vi "SeCrTs-RD DI Indexing dis.vi"() -> ()   [LabVIEW 2022 SP3]
panel:
  in  "DI CONFIG":T1
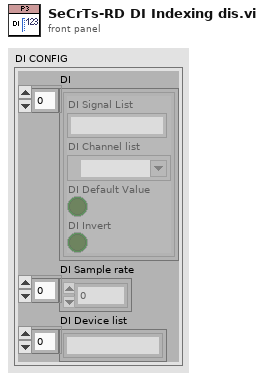
[diagram p1: front panel]
types:
  T1 = cluster{"DI":cluster{"DI Signal List":string, "DI Channel list":tag, "DI Default Value":bool, "DI Invert":bool}[], "DI Sample rate":i32[], "DI Device list  ":string[]}
  T2 = cluster{"DI Signal List":string, "DI Channel list":tag, "DI Default Value":bool, "DI Invert":bool}[]
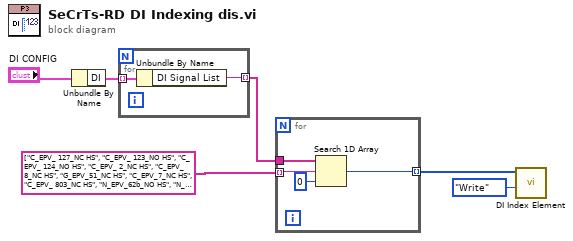
[diagram p0: block diagram]
diagram:
  n1 = Unbundle By Name("DI CONFIG") -> ("DI"=w5:T2)
  n2 = for {
    tunnel: [w8] -> w6 mode=indexing
    tunnel: w5 -> [w7] mode=indexing
    n3 = Unbundle By Name(w7) -> ("DI Signal List"=w8:string)
  }
  n4 = for {
    tunnel: w6 -> [w12]
    tunnel: string[] ["C_EPV_ 127_NC HS", "C_EPV_ 123_NO HS", "C_EPV_ 124_NO HS", "C_EPV_ 2_NC HS", "C_EPV_ 8_NC HS", "G_EPV_51_NC HS", "C_EPV_7_NC HS", "C_EPV_ 803_NC HS", "N_EPV_62b_NO HS", "N_EPV_62a_NO HS", "N_EPV_61_NO HS", "C_EPV_ 141_NO HS", "C_EPV_16_NC HS", "C_EPV_18_NO HS", "F_EPV_1352_NO HS", "N_EPV_202_NO HS", "N_EPV_203_NO HS", "F_EPV_136 _NC HS", "N_EPV_68_NO HS", "F_EPV_28_NC HS", "F_EPV_132_NO HS", "N_EPV_69_NO HS", "N_EPV_142_NO HS", "F_EPV_131_NO HS", "F_EPV_21_NC HS", "F_EPV_41_NC HS", "N_EPV_206_NO HS", "N_EPV_75_NO HS", "F_EPV_33_NC HS"] -> [w11] mode=indexing
    tunnel: [w9] -> w3 mode=indexing
    n5 = Search 1D Array(1D array=w12, element=w11, start index (0)=0) -> (index of element=w9:i32)
  }
  n6 = call "DI Index Element.vi"("Write/Read"=enum16{"Write", "Read"}."Write", "Index Element"=w3) -> ()  [unwired: 9 in, 1 out]
